vi "PoseAndTargeting.vi"() -> ()   [LabVIEW 2020]
doc: "Manages the robot's pose (position, heading, and velocity) and targeting information. Data from the IMU, swerve drive encoders, swerve azimuth encoders, turret enoder, and LimeLight are fused together to estimate these values. Supports pose resets on boot, from the Autonomous Sequencer, and on command from the FRC 4265 Dashboard."
uses:
  c71665c3-219d-469c-9b81-2f0818bb1921.vi
  GlobalDriverStationData.vi
  GlobalDrivebase.vi
panel:
  in  "Close Acceptable Heading Error (deg)":dbl=5.0
  in  "Radial Target Shift (in)":dbl
  in  "Angular Target Shift (deg)":dbl
  in  "Min Timed Aligned (ms)":u32=100
  in  "Far Acceptable Heading Error (deg)":dbl=3.0
  in  "Vision Trust Threshold (in)":dbl=5.0
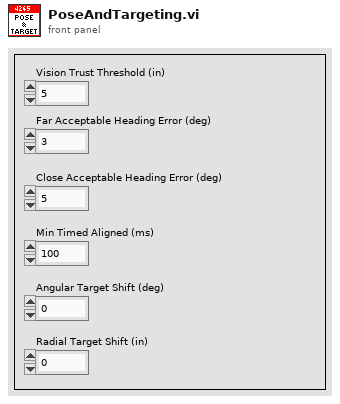
[diagram p1: front panel]
types:
  T1 = enum16{"Normal", "Auto Set", "Reset IMU", "Manual Push", "Init"}
  T2 = enum16{"Center", "North", "NorthWest", "West", "SouthWest", "South", "SouthEast", "East", "NorthEast"}
  T3 = cluster{"Transitioning":bool, "Position (in)":dbl, "Velocity (ft/s)":dbl, "Azimuth Position (deg) [-180,+180]":dbl}
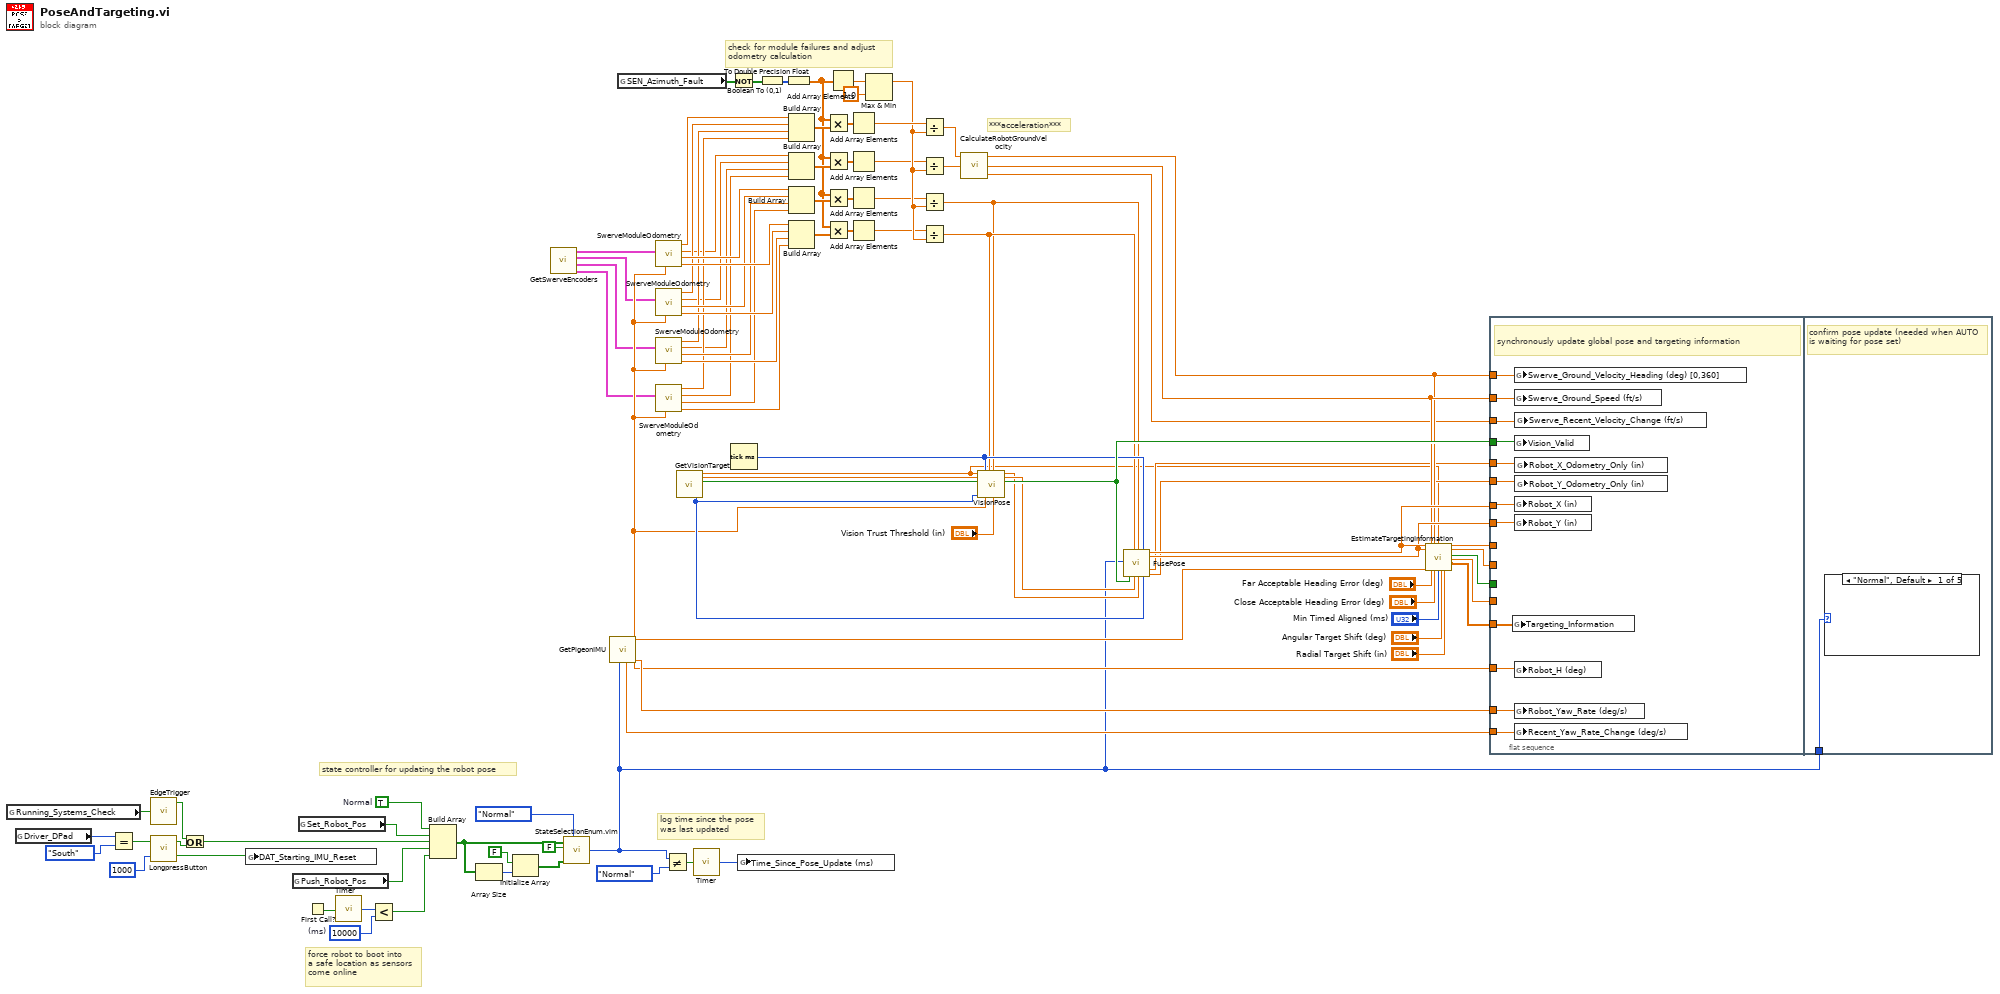
[diagram p0: block diagram]
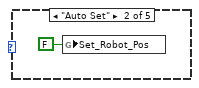
[diagram p2: hidden frame]
diagram:
  w86 = u32 10000  # (ms)
  w92 = TRUE  # Normal
  # "***acceleration***"
  # "force robot to boot into\na safe location as sensors\ncome online"
  # "log time since the pose\nwas last updated"
  # "state controller for updating the robot pose"
  # "check for module failures and adjust\nodometry calculation"
  n1 = global read "GlobalDriverStationData.vi" "Running_Systems_Check"() -> (w29:bool)
  n2 = global read "GlobalDriverStationData.vi" "Driver_DPad"() -> (w73:T2)
  n3 = Equal?(x=w73, y=T2."South") -> (x = y?=w72:bool)
  n4 = call "EdgeTrigger.vi"("Input Signal"=w29) -> ("Rising Edge Trigger"=w27:bool)  [unwired: 2 out]
  n5 = call "LongpressButton.vi"("Threshold (ms)"=u32 1000, "Button"=w72) -> ("Starting Press"=w25:bool, "Longpress Button"=w28:bool)
  n6 = Or(x=w27, y=w28) -> (x .or. y?=w26:bool)
  n7 = global write "GlobalDrivebase.vi" "DAT_Starting_IMU_Reset"(w25) -> ()
  n8 = global read "GlobalPoseAndTargeting.vi" "Push_Robot_Pos"() -> (w93:bool)
  n9 = global read "GlobalPoseAndTargeting.vi" "Set_Robot_Pos"() -> (w85:bool)
  n10 = First Call?() -> (First Call?: T/F=w89:bool)
  n11 = call "Timer.vi"("Reset Timer"=w89) -> ("Time (ms)"=w88:u32)
  n12 = Less?(x=w88, y=w86) -> (x < y?=w87:bool)
  n13 = Build Array(w92, w85, w26, w93, w87) -> (w67:bool[])
  n14 = Array Size(array=w67) -> (size(s)=w70:i32)
  n15 = Initialize Array(FALSE, w70) -> (w66:bool[])
  n16 = call "GetSwerveEncoders.vi"() -> ("Swerve 3 Encoder Data"=w21:T3, "Swerve 2 Encoder Data"=w22:T3, "Swerve 1 Encoder Data"=w23:T3, "Swerve 0 Encoder Data"=w24:T3)  [unwired: 5 in]
  n17 = call "StateSelectionEnum.vim"("Enum Def"=T1."Normal", "Disallowed States"=w66, "Enable Edge Trigger"=FALSE, "State Triggers"=w67) -> ("Selected State"=w30:T1)  [unwired: 1 in, 1 out]
  n18 = call "GetPigeonIMU.vi"("Pose Mode"=w30) -> ("Yaw Rate (deg/s)"=w44:dbl, "Yaw (deg)"=w31:dbl, "Recent Yaw Rate Change (deg/s)"=w35:dbl)  [unwired: 8 in]
  n19 = global read "GlobalDrivebase.vi" "SEN_Azimuth_Fault"() -> (w11:bool[])
  n20 = call "SwerveModuleOdometry.vi"("Robot Heading(deg)"=w31, "Swerve Encoder Data"=w24) -> ("Delta Y (in)"=w95:dbl, "Delta X (in)"=w84:dbl, "Velocity Y (ft/s)"=w77:dbl, "Velocity X (ft/s)"=w18:dbl)  [unwired: 4 in]
  n21 = call "SwerveModuleOdometry.vi"("Robot Heading(deg)"=w31, "Swerve Encoder Data"=w23) -> ("Delta Y (in)"=w96:dbl, "Delta X (in)"=w83:dbl, "Velocity Y (ft/s)"=w76:dbl, "Velocity X (ft/s)"=w80:dbl)  [unwired: 4 in]
  n22 = call "SwerveModuleOdometry.vi"("Robot Heading(deg)"=w31, "Swerve Encoder Data"=w22) -> ("Delta Y (in)"=w97:dbl, "Delta X (in)"=w82:dbl, "Velocity Y (ft/s)"=w75:dbl, "Velocity X (ft/s)"=w79:dbl)  [unwired: 4 in]
  n23 = call "SwerveModuleOdometry.vi"("Robot Heading(deg)"=w31, "Swerve Encoder Data"=w21) -> ("Delta Y (in)"=w98:dbl, "Delta X (in)"=w81:dbl, "Velocity Y (ft/s)"=w74:dbl, "Velocity X (ft/s)"=w78:dbl)  [unwired: 4 in]
  n24 = Not Equal?(x=w30, y=T1."Normal") -> (x != y?=w91:bool)
  n25 = call "GetVisionTarget.vi"() -> ("Vision Timestamp (ms)"=w43:u32, "Vision Horizontal Angle to Target (deg) [t-?]"=w33:dbl, "Vision Vertical Angle to Target (deg) [t-?]"=w57:dbl, "Vision Target Valid [t-?]"=w56:bool)  [unwired: 16 in]
  n26 = call "Timer.vi"("Reset Timer"=w91) -> ("Time (ms)"=w90:u32)
  n27 = Not(x=w11) -> (.not. x?=w20:bool[])
  n28 = Tick Count (ms)() -> (millisecond timer value=w42:u32)
  n29 = global write "GlobalPoseAndTargeting.vi" "Time_Since_Pose_Update (ms)"(w90) -> ()
  n30 = Boolean To (0,1)(Boolean=w20) -> (0, 1=w19:i16[])
  n31 = To Double Precision Float(number=w19) -> (double precision float=w2:dbl[])
  n32 = Build Array(w18, w80, w79, w78) -> (w12:dbl[])
  n33 = Build Array(w77, w76, w75, w74) -> (w9:dbl[])
  n34 = Build Array(w84, w83, w82, w81) -> (w6:dbl[])
  n35 = Build Array(w95, w96, w97, w98) -> (w3:dbl[])
  n36 = Multiply(x=w2, y=w12) -> (x*y=w17:dbl[])
  n37 = Multiply(x=w2, y=w9) -> (x*y=w10:dbl[])
  n38 = Multiply(x=w2, y=w6) -> (x*y=w7:dbl[])
  n39 = Multiply(x=w2, y=w3) -> (x*y=w4:dbl[])
  n40 = Add Array Elements(numeric array=w2) -> (sum=w15:dbl)
  n41 = Add Array Elements(numeric array=w17) -> (sum=w16:dbl)
  n42 = Add Array Elements(numeric array=w10) -> (sum=w8:dbl)
  n43 = Add Array Elements(numeric array=w7) -> (sum=w5:dbl)
  n44 = Add Array Elements(numeric array=w4) -> (sum=w1:dbl)
  n45 = Max & Min(x=w15, y=1.0) -> (max(x,y)=w13:dbl)  [unwired: 1 out]
  n46 = Divide(x=w16, y=w13) -> (x/y=w51:dbl)
  n47 = Divide(x=w8, y=w13) -> (x/y=w52:dbl)
  n48 = Divide(x=w5, y=w13) -> (x/y=w38:dbl)
  n49 = Divide(x=w1, y=w13) -> (x/y=w39:dbl)
  n50 = call "CalculateRobotGroundVelocity.vi"("Velocity Y (ft/s)"=w52, "Velocity X (ft/s)"=w51) -> ("Recent Velocity Change (ft/s)"=w36:dbl, "Velocity Magnitude (ft/s)"=w46:dbl, "Velocity Heading (deg)"=w45:dbl)  [unwired: 1 in]
  n51 = call "VisionPose.vi"("Vision Horizontal Angle to Target (deg) [t-?]"=w33, "Vision Vertical Angle to Target (deg) [t-?]"=w57, "Vision Target Valid [t-?]"=w56, "Vision Timestamp (ms)"=w43, "Odometry Timestamp (ms)"=w42, "Robot Heading (deg) [t0]"=w31, "Odometry Delta Y (in) [t0]"=w39, "Odometry Delta X (in) [t0]"=w38, "Vision Trust Threshold (in)"="Vision Trust Threshold (in)") -> ("Vision X (in) [t-?]"=w53:dbl, "Vision Y (in) [t-?]"=w54:dbl, "Vision Valid [t-?]"=w55:bool)  [unwired: 8 in]
  n52 = call "FusePose.vi"("Pose Mode"=w30, "Vision Valid [t-?]"=w55, "Odometry Delta Y (in) [t0]"=w39, "Vision Y (in) [t-?]"=w54, "Odometry Delta X (in) [t0]"=w38, "Vision X (in) [t-?]"=w53, "Odometry Timestamp (ms)"=w42, "Vision Timestamp (ms)"=w43) -> ("X (in) [t0]"=w60:dbl, "Y (in) [t0]"=w59:dbl, "X Odometry Only (in) [t0]"=w41:dbl, "Y Odometry Only (in) [t0]"=w40:dbl)  [unwired: 8 in]
  n53 = call "EstimateTargetingInformation.vi"("X (in) [t0]"=w60, "Y (in) [t0]"=w59, "Robot Heading (deg)"=w31, "Velocity Magnitude (ft/s)"=w46, "Far Acceptable Heading Error (deg)"="Far Acceptable Heading Error (deg)", "Velocity Heading (deg)"=w45, "Close Acceptable Heading Error (deg)"="Close Acceptable Heading Error (deg)", "Vision Horizontal Angle to Target (deg) [t-?]"=w33, "Min Timed Aligned (ms)"="Min Timed Aligned (ms)", "Angular Target Shift (deg)"="Angular Target Shift (deg)", "Radial Target Shift (in)"="Radial Target Shift (in)") -> ("Fused Distance to Target (in)"=w63:dbl, "Fused Heading to Target (deg)"=w62:dbl, "Pointed At Target"=w61:bool, "Pointing Angle Error (deg)"=w50:dbl, "Targeting Predictions"=w47:dbl[])  [unwired: 12 in]
  n54 = flat-sequence {
    tunnel: w31 -> [w110]
    tunnel: w63 -> [_]
    tunnel: w62 -> [_]
    tunnel: w61 -> [_]
    tunnel: w60 -> [w109]
    tunnel: w59 -> [w108]
    tunnel: w55 -> [w107]
    tunnel: w50 -> [_]
    tunnel: w46 -> [w106]
    tunnel: w45 -> [w105]
    tunnel: w47 -> [w104]
    tunnel: w44 -> [w103]
    tunnel: w41 -> [w102]
    tunnel: w40 -> [w101]
    tunnel: w36 -> [w100]
    tunnel: w35 -> [w99]
    tunnel: w30 -> [w111]
    frame #0 {
      # "synchronously update global pose and targeting information"
      n55 = global write "GlobalPoseAndTargeting.vi" "Targeting_Information"(w104) -> ()
      n56 = global write "GlobalPoseAndTargeting.vi" "Swerve_Ground_Velocity_Heading (deg) [0,360]"(w105) -> ()
      n57 = global write "GlobalPoseAndTargeting.vi" "Swerve_Ground_Speed (ft/s)"(w106) -> ()
      n58 = global write "GlobalPoseAndTargeting.vi" "Vision_Valid"(w107) -> ()
      n59 = global write "GlobalPoseAndTargeting.vi" "Robot_X (in)"(w109) -> ()
      n60 = global write "GlobalPoseAndTargeting.vi" "Robot_Y (in)"(w108) -> ()
      n61 = global write "GlobalPoseAndTargeting.vi" "Robot_H (deg)"(w110) -> ()
      n62 = global write "GlobalPoseAndTargeting.vi" "Robot_Yaw_Rate (deg/s)"(w103) -> ()
      n63 = global write "GlobalPoseAndTargeting.vi" "Recent_Yaw_Rate_Change (deg/s)"(w99) -> ()
      n64 = global write "GlobalPoseAndTargeting.vi" "Swerve_Recent_Velocity_Change (ft/s)"(w100) -> ()
      n65 = global write "GlobalPoseAndTargeting.vi" "Robot_X_Odometry_Only (in)"(w102) -> ()
      n66 = global write "GlobalPoseAndTargeting.vi" "Robot_Y_Odometry_Only (in)"(w101) -> ()
    }
    frame #1 {
      # "confirm pose update (needed when AUTO is waiting for pose set)"
      n67 = case shown="\"Normal\", Default" w111 {
        frame "Normal", Default {
        }
        frame "Auto Set" {
          n68 = global write "GlobalPoseAndTargeting.vi" "Set_Robot_Pos"(FALSE ("Set_Robot_Pos")) -> ()
        }
        frame "Reset IMU" {
        }
        frame "Manual Push" {
        }
        frame "Init" {
        }
      }
    }
  }
